vi "Periodic Task Hopper Control.vi"(8 "error in":errorcluster) -> ()   [LabVIEW 2016]
doc: "This VI runs in parallel to other tasks. It can contain as many user-defined periodic loops as you need. These can carry out PID or other sorts of timed response."
uses:
  Robot Global Data.vi
  HopperStates.ctl
  <vilib>/Rock Robotics/WPI/SafetyOutput/WPI_SafetyOutputConfigMenu.ctl
panel:
  in  "HighAutoDownSpeed":dbl=0.15
  in  "LowAutoDownSpeed":dbl=-0.15
  in  "HighAutoUpSpeed":dbl=-0.1
  in  "LowAutoUpSpeed":dbl=0.1
  in  "HighManualDownSpeed":dbl=0.15
  in  "LowManualDownSpeed":dbl=-0.15
  in  "HighManualUpSpeed":dbl=-0.1
  in  "LowManualUpSpeed":dbl=0.1
  in  "HighHopperMotorSpeed":dbl
  in  "LowHopperMotorSpeed":dbl
  in  "LDPhotoeyeOffTimerLimit":u32=200
  in  "LDPhotoeyeOnTimerLimit":u32=300
  in  "LDStartTimeOff":u32
  in  "LDPhotoeyeOnTimerDone":bool
  in  "LDStartTimeOn":u32
  in  "LDPhotoeyeOnTiming":bool
  in  "LDPhotoeyeOffTiming":bool
  in  "LUPhotoeyeOffTimerLimit":u32=200
  in  "LUPhotoeyeOnTimerLimit":u32=300
  in  "LUStartTimeOff":u32
  in  "LUPhotoeyeOnTimerDone":bool
  in  "LUStartTimeOn":u32
  in  "LUPhotoeyeOnTiming":bool
  in  "LUPhotoeyeOffTiming":bool
  in  "HDPhotoeyeOffTimerLimit":u32=200
  in  "HDPhotoeyeOnTimerLimit":u32=300
  in  "HDStartTimeOff":u32
  in  "HDPhotoeyeOnTimerDone":bool
  in  "HDStartTimeOn":u32
  in  "HDPhotoeyeOnTiming":bool
  in  "HDPhotoeyeOffTiming":bool
  in  "HUPhotoeyeOffTimerLimit":u32=200
  in  "HUPhotoeyeOnTimerLimit":u32=300
  in  "HUStartTimeOff":u32
  in  "HUPhotoeyeOnTimerDone":bool
  in  "HUStartTimeOn":u32
  in  "HUPhotoeyeOnTiming":bool
  in  "HUPhotoeyeOffTiming":bool
  # "High Side Up Photoeye"
  # "High Side Down Photoeye"
  # "Current Motor Speed"
  # "Manual Control Speed Settings"
  # "Low Side Up Photoeye"
  # "Low Side Down Photoeye"
  # "Automatic Control Speed Settings"
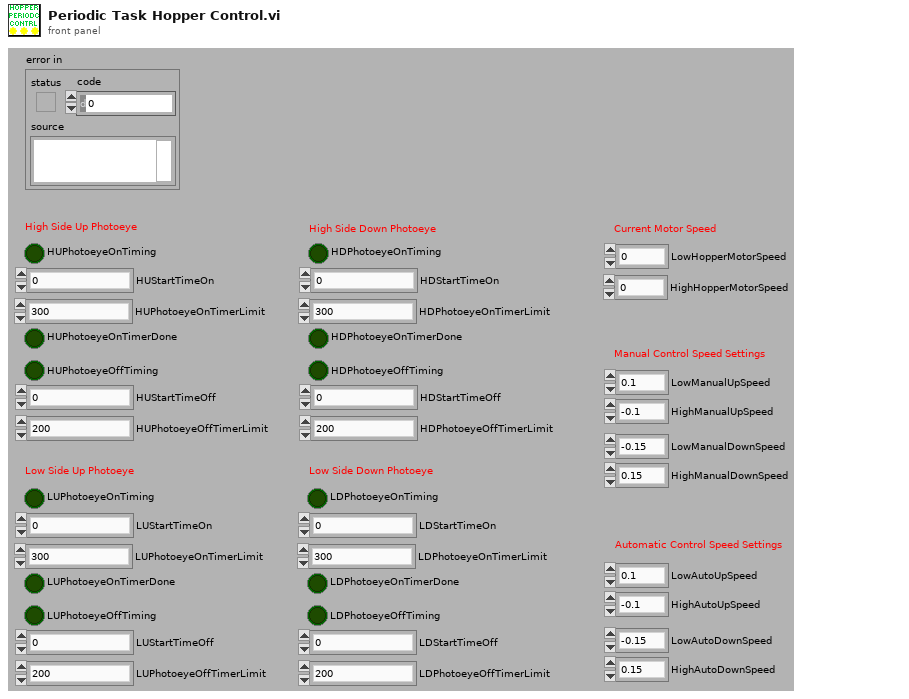
[diagram p1: front panel]
types:
  T1 = typedef "WPI_SafetyOutputConfigMenu.ctl" = enum16{"Enable", "Disable"}
  T2 = typedef "HopperStates.ctl" = enum16{"HopperIdle", "ManualRaiseHopper", "ManualLowerHopper", "AutoRaiseHopper", "AutoLowerHopper", "AtTop", "AtBottom"}
  T3 = typedef "WPI_MotorControlDeviceRef.ctl" = cluster{"DeviceStatus":errorcluster, "Type":T4, "PWM":cluster{"PWM Channel":T5, "DeadBand":T6}, "CAN":cluster{"Device Number":u8, "SetOutput VI Ref":variant, "GetOutput VI Ref":variant, "Enable VI Ref":variant, "Disable VI Ref":variant, "Data":variant}, "Invert":bool}
  T4 = typedef "WPI_MotorControlType.ctl" = enum16{"PWM", "CAN"}
  T5 = typedef "FPGA_DIOPWMChannel.ctl" = enum8{"PWM 0", "PWM 1", "PWM 2", "PWM 3", "PWM 4", "PWM 5", "PWM 6", "PWM 7", "PWM 8", "PWM 9", "PWM MXP 0", "PWM MXP 1", "PWM MXP 2", "PWM MXP 3", "PWM MXP 4", "PWM MXP 5", "PWM MXP 6", "PWM MXP 7", "PWM MXP 8", "PWM MXP 9", "Invalid"}
  T6 = typedef "WPI_PWMDeadband.ctl" = cluster{"Name":string, "maxPositivePwm":i32, "minPositivePwm":i32, "centerPwm":i32, "maxNegativePwm":i32, "minNegativePwm":i32, "angularRange":u16}
  T7 = typedef "WPI_DigitalInputDevRef.ctl" = cluster{"DevStatus":errorcluster, "DIO Channel":T8}
  T8 = typedef "FPGA_DIOChannel.ctl" = enum8{"DIO 0", "DIO 1", "DIO 2", "DIO 3", "DIO 4", "DIO 5", "DIO 6", "DIO 7", "DIO 8", "DIO 9", "DIO MXP 0", "DIO MXP 1", "DIO MXP 2", "DIO MXP 3", "DIO MXP 4", "DIO MXP 5", "DIO MXP 6", "DIO MXP 7", "DIO MXP 8", "DIO MXP 9", "DIO MXP 10", "DIO MXP 11", "DIO MXP 12", "DIO MXP 13", "DIO MXP 14", "DIO MXP 15", "SPI Port CS1", "SPI Port CS2", "SPI Port CS3", "SPI Port MISO", "SPI Port MOSI", "Invalid"}
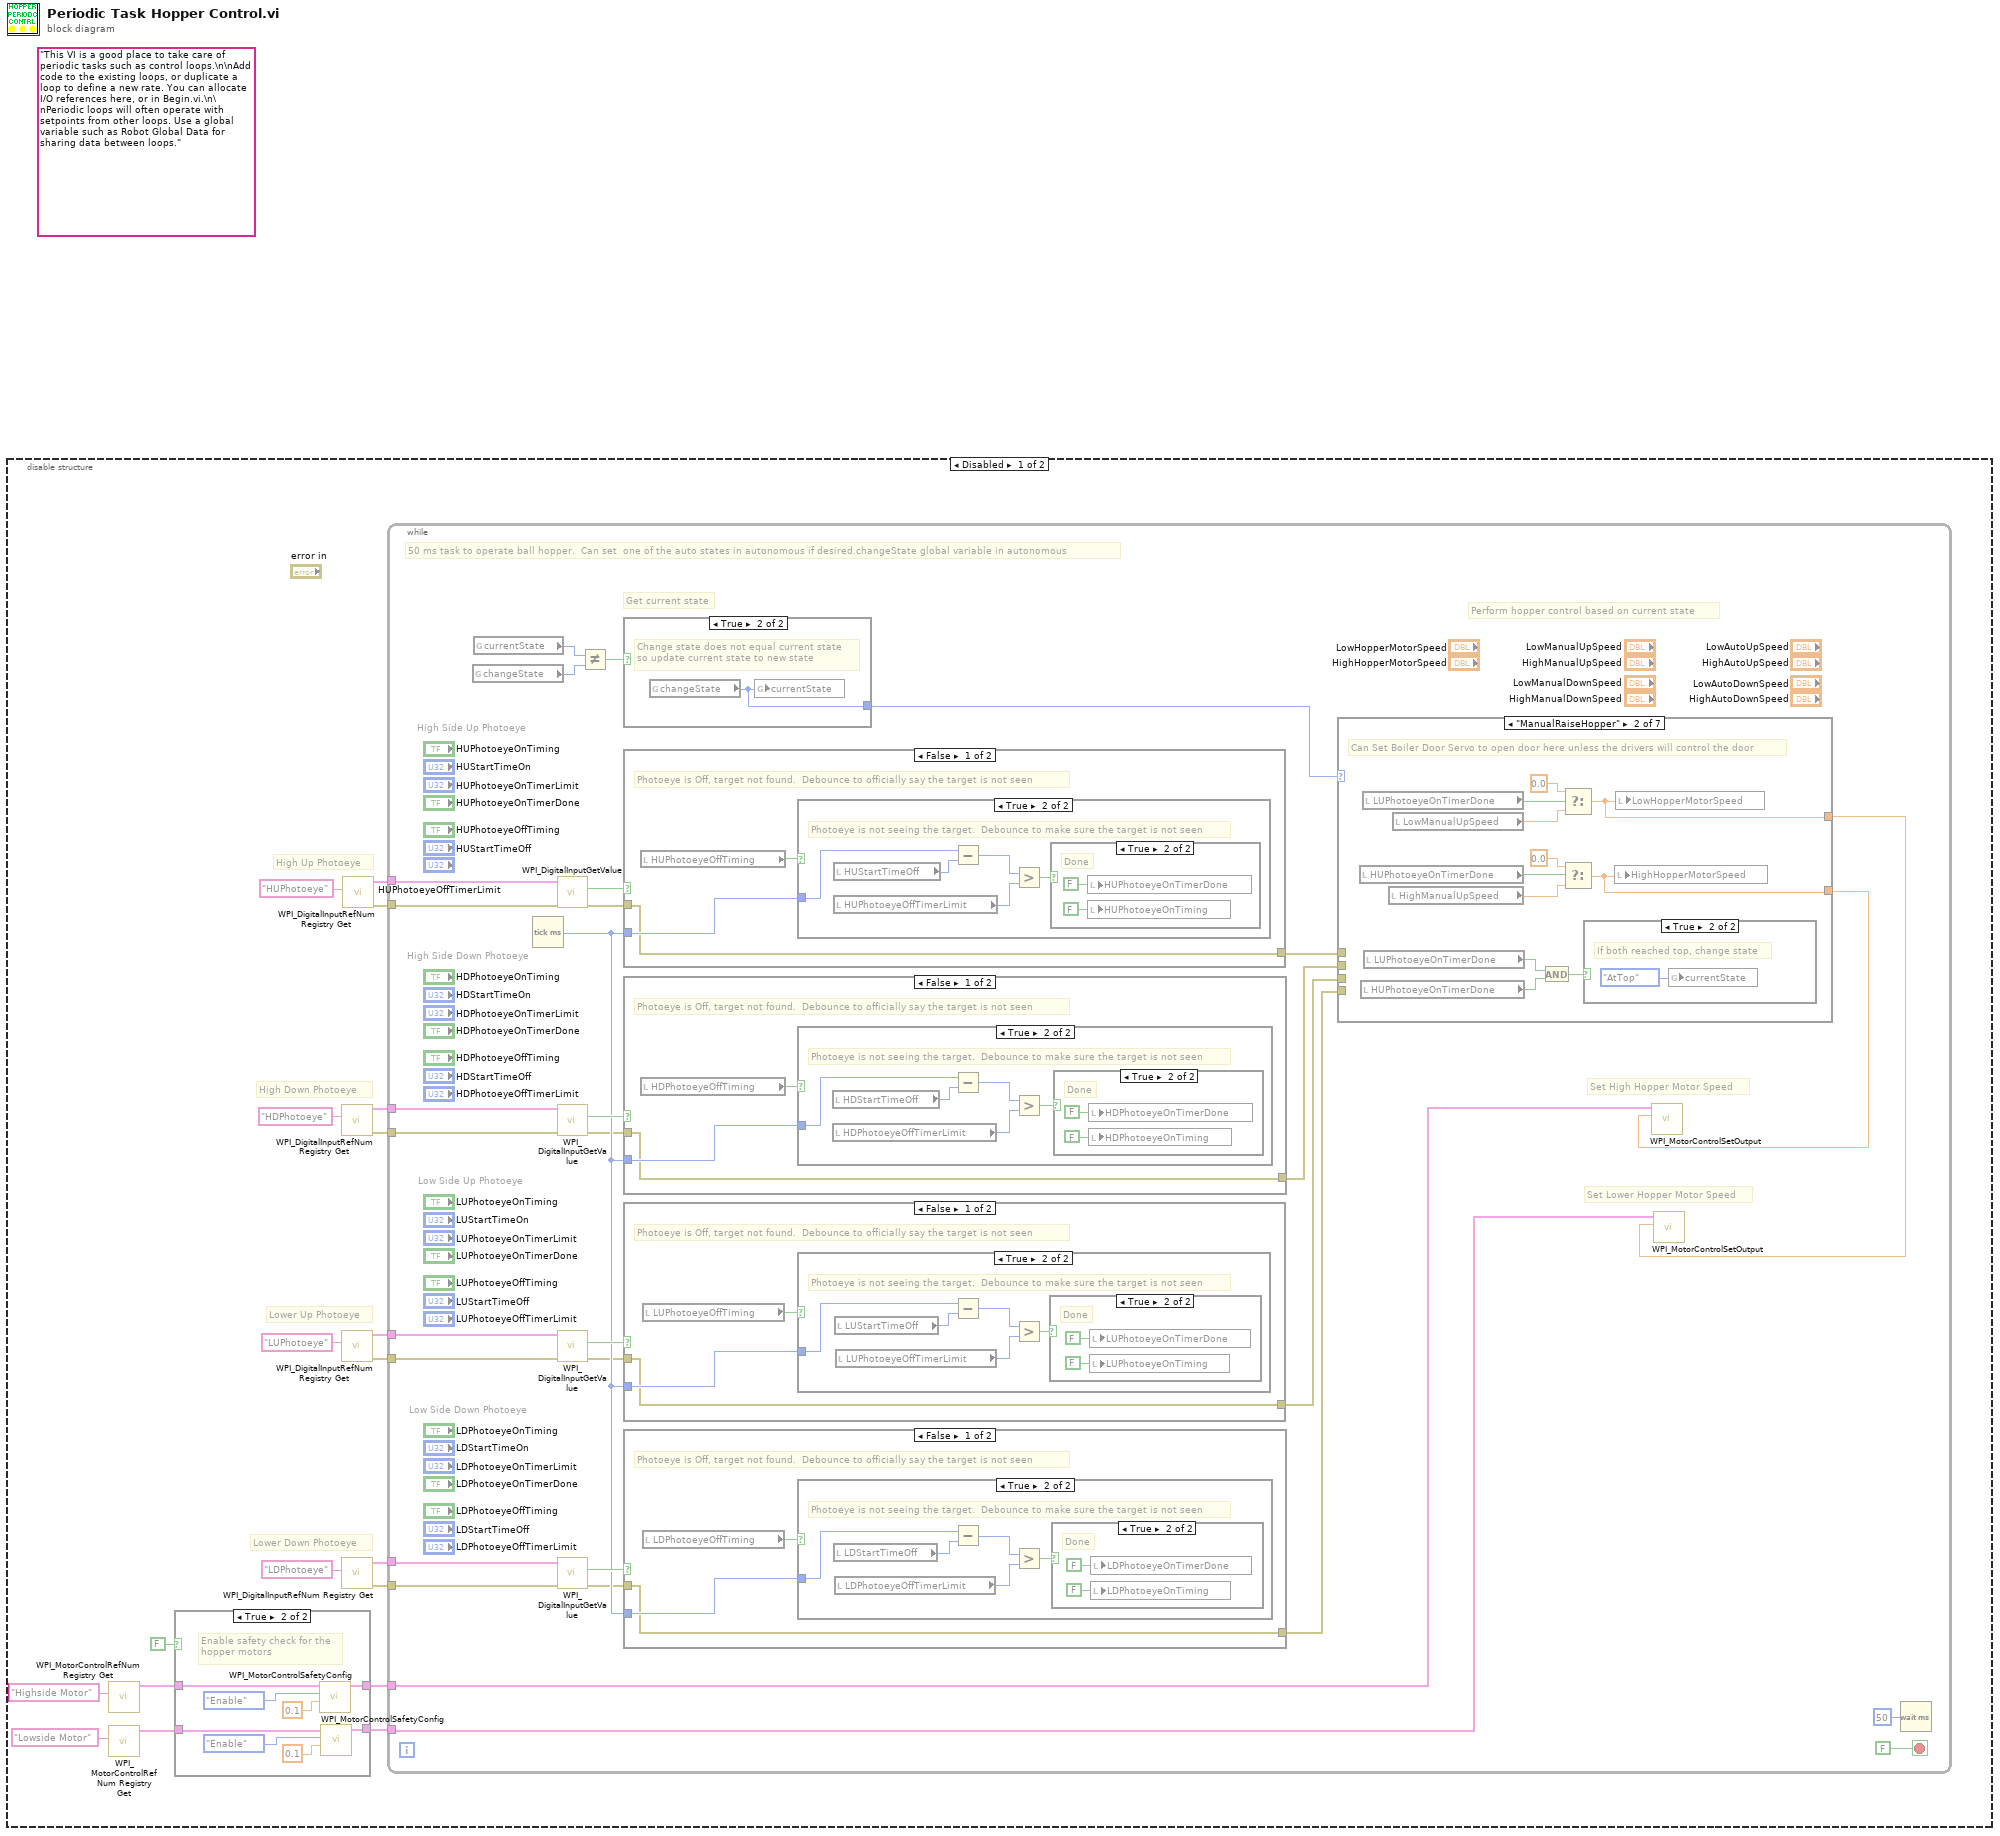
[diagram p0: block diagram]
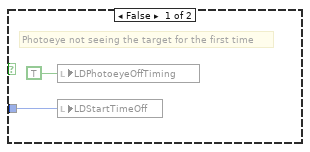
[diagram p3: hidden frame]
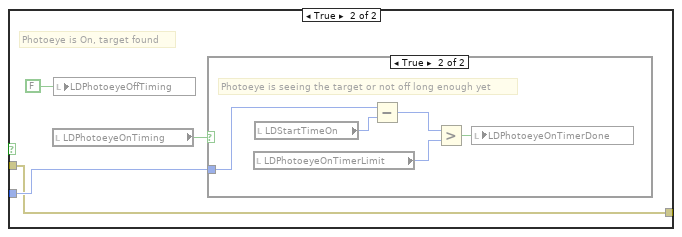
[diagram p5: hidden frame]
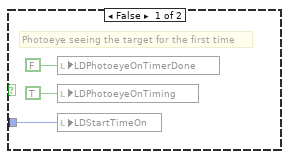
[diagram p6: hidden frame]
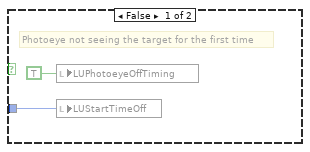
[diagram p7: hidden frame]
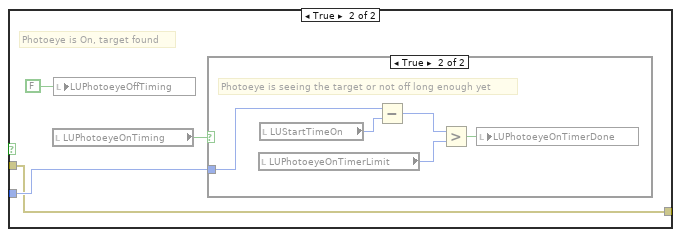
[diagram p9: hidden frame]
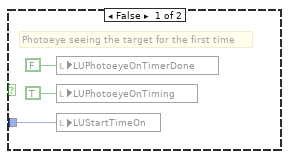
[diagram p10: hidden frame]
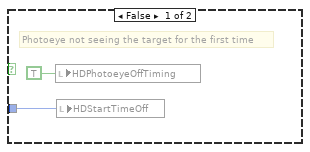
[diagram p11: hidden frame]
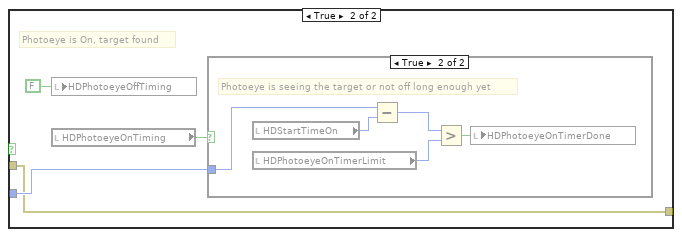
[diagram p13: hidden frame]
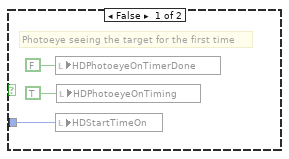
[diagram p14: hidden frame]
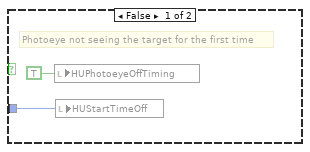
[diagram p15: hidden frame]
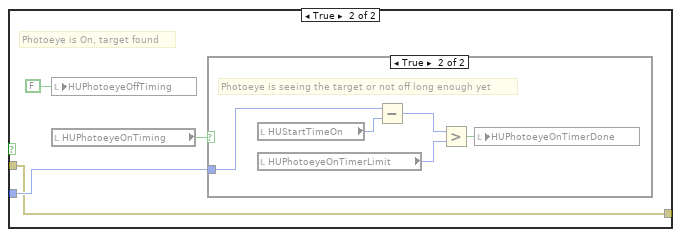
[diagram p17: hidden frame]
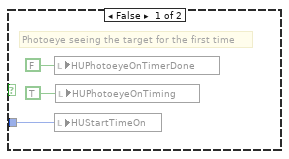
[diagram p18: hidden frame]
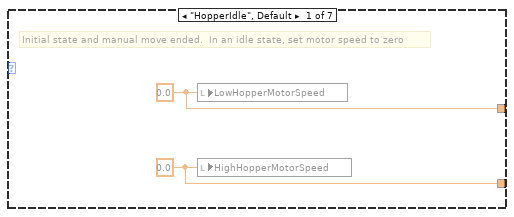
[diagram p19: hidden frame]
diagram:
  (unwired) "This VI is a good place to take care of periodic tasks such as control loops.\n\nAdd code to the existing loops, or duplicate a loop to define a new rate. You can allocate I/O references here, or in Begin.vi.\n\nPeriodic loops will often operate with setpoints from other loops. Use a global variable such as Robot Global Data for sharing data between loops."
  n1 = disable-structure shown="Disabled" {
    frame Disabled {
      # "Lower Down Photoeye"
      # "Lower Up Photoeye"
      # "High Down Photoeye"
      # "High Up Photoeye"
      n2 = call <vilib>:"WPI_MotorControlRefNum Registry Get.vi"("refnum name"="Highside Motor") -> ("MotorControlDevRef"=w5:T3)  [unwired: 9 in, 1 out]
      n3 = call <vilib>:"WPI_MotorControlRefNum Registry Get.vi"("refnum name"="Lowside Motor") -> ("MotorControlDevRef"=w3:T3)  [unwired: 9 in, 1 out]
      n4 = case shown="True" FALSE {
        tunnel: w5 -> [w21 w29]
        tunnel: [w21 w28] -> w4
        tunnel: w3 -> [w20 w27]
        tunnel: [w20 w26] -> w2
        frame False {
          # "Skip safety check since this\nVI loop should never be\nstarved"
        }
        frame True {
          # "Enable safety check for the\nhopper motors"
          n5 = call <vilib>:"WPI_MotorControlSafetyConfig.vi"("timeout (s)"=0.1, "mode"=WPI_SafetyOutputConfigMenu."Enable", "MotorControlDevRef"=w29) -> ("MotorControlDevRef"=w28:T3)  [unwired: 7 in, 1 out]
          n6 = call <vilib>:"WPI_MotorControlSafetyConfig.vi"("timeout (s)"=0.1, "mode"=WPI_SafetyOutputConfigMenu."Enable", "MotorControlDevRef"=w27) -> ("MotorControlDevRef"=w26:T3)  [unwired: 7 in, 1 out]
        }
      }
      n7 = call <vilib>:"WPI_DigitalInputRefNum Registry Get.vi"("refnum name"="HDPhotoeye") -> ("error out"=w8:errorcluster, "DigitalInputDevRef"=w9:T7)  [unwired: 9 in]
      n8 = call <vilib>:"WPI_DigitalInputRefNum Registry Get.vi"("refnum name"="LUPhotoeye") -> ("error out"=w10:errorcluster, "DigitalInputDevRef"=w11:T7)  [unwired: 9 in]
      n9 = call <vilib>:"WPI_DigitalInputRefNum Registry Get.vi"("refnum name"="LDPhotoeye") -> ("error out"=w12:errorcluster, "DigitalInputDevRef"=w13:T7)  [unwired: 9 in]
      n10 = call <vilib>:"WPI_DigitalInputRefNum Registry Get.vi"("refnum name"="HUPhotoeye") -> ("error out"=w17:errorcluster, "DigitalInputDevRef"=w18:T7)  [unwired: 9 in]
      n11 = while {
        tunnel: w18 -> [w41]
        tunnel: w17 -> [w40]
        tunnel: w9 -> [w39]
        tunnel: w8 -> [w38]
        tunnel: w11 -> [w37]
        tunnel: w10 -> [w36]
        tunnel: w13 -> [w35]
        tunnel: w12 -> [w34]
        tunnel: w2 -> [w30]
        tunnel: w4 -> [w31]
        stop <- FALSE stop-if-true
        # "Low Side Down Photoeye"
        # "Low Side Up Photoeye"
        # "High Side Down Photoeye"
        # "High Side Up Photoeye"
        # "Set Lower Hopper Motor Speed"
        # "Set High Hopper Motor Speed"
        # "Get current state"
        # "Perform hopper control based on current state"
        # "50 ms task to operate ball hopper.  Can set  one of the auto states in autonomous if desired.changeState global variable in autonomous"
        n12 = global read "Robot Global Data.vi" "changeState"() -> (w57:T2)
        n13 = global read "Robot Global Data.vi" "currentState"() -> (w58:T2)
        n14 = Tick Count (ms)() -> (millisecond timer value=w50:u32)
        n15 = call <vilib>:"WPI_DigitalInputGetValue.vi"("error in (no error)"=w40, "DigitalInputDevRef"=w41) -> ("error out"=w48:errorcluster, "Value"=w54:bool)  [unwired: 7 in, 1 out]
        n16 = call <vilib>:"WPI_DigitalInputGetValue.vi"("error in (no error)"=w38, "DigitalInputDevRef"=w39) -> ("error out"=w47:errorcluster, "Value"=w53:bool)  [unwired: 7 in, 1 out]
        n17 = call <vilib>:"WPI_DigitalInputGetValue.vi"("error in (no error)"=w36, "DigitalInputDevRef"=w37) -> ("error out"=w46:errorcluster, "Value"=w52:bool)  [unwired: 7 in, 1 out]
        n18 = call <vilib>:"WPI_DigitalInputGetValue.vi"("error in (no error)"=w34, "DigitalInputDevRef"=w35) -> ("error out"=w49:errorcluster, "Value"=w51:bool)  [unwired: 7 in, 1 out]
        n19 = Not Equal?(x=w58, y=w57) -> (x != y?=w56:bool)
        n20 = case shown="True" w56 {
          tunnel: [w211 w212] -> w55
          frame False {
            # "Change state equals current state \nso keep current state"
            n21 = global read "Robot Global Data.vi" "currentState"() -> (w211:T2)
          }
          frame True {
            # "Change state does not equal current state \nso update current state to new state"
            n22 = global read "Robot Global Data.vi" "changeState"() -> (w212:T2)
            n23 = global write "Robot Global Data.vi" "currentState"(w212) -> ()
          }
        }
        n24 = case shown="False" w54 {
          tunnel: w50 -> [w134 w146]
          tunnel: w48 -> [w133 w145]
          tunnel: [w133 w145] -> w45
          frame False {
            # "Photoeye is Off, target not found.  Debounce to officially say the target is not seen"
            n25 = local read "HUPhotoeyeOffTiming"() -> (w135:bool)
            n26 = case shown="True" w135 {
              tunnel: w134 -> [w137 w141]
              frame False {
                # "Photoeye not seeing the target for the first time"
                n27 = local write "HUPhotoeyeOffTiming"(TRUE ("PhotoeyeOffTiming")) -> ()
                n28 = local write "HUStartTimeOff"(w137) -> ()
              }
              frame True {
                # "Photoeye is not seeing the target.  Debounce to make sure the target is not seen"
                n29 = local read "HUStartTimeOff"() -> (w140:u32)
                n30 = local read "HUPhotoeyeOffTimerLimit"() -> (w139:u32)
                n31 = Subtract(x=w141, y=w140) -> (x-y=w142:u32)
                n32 = Greater?(x=w142, y=w139) -> (0:w138:bool)
                n33 = case shown="True" w138 {
                  frame False {
                    # "Waiting for Off to time out"
                  }
                  frame True {
                    # "Done"
                    n34 = local write "HUPhotoeyeOnTimerDone"(FALSE ("HUPhotoeyeOnTimerDone")) -> ()
                    n35 = local write "HUPhotoeyeOnTiming"(FALSE ("HUPhotoeyeOnTiming")) -> ()
                  }
                }
              }
            }
          }
          frame True {
            # "Photoeye is On, target found"
            n36 = local write "HUPhotoeyeOffTiming"(FALSE ("PhotoeyeOffTiming")) -> ()
            n37 = local read "HUPhotoeyeOnTiming"() -> (w147:bool)
            n38 = case shown="True" w147 {
              tunnel: w146 -> [w151 w156]
              frame False {
                # "Photoeye seeing the target for the first time"
                n39 = local write "HUPhotoeyeOnTimerDone"(FALSE ("PhotoeyeOnTimerDone")) -> ()
                n40 = local write "HUStartTimeOn"(w151) -> ()
                n41 = local write "HUPhotoeyeOnTiming"(TRUE ("PhotoeyeOnTiming")) -> ()
              }
              frame True {
                # "Photoeye is seeing the target or not off long enough yet"
                n42 = local read "HUStartTimeOn"() -> (w155:u32)
                n43 = local read "HUPhotoeyeOnTimerLimit"() -> (w153:u32)
                n44 = Subtract(x=w156, y=w155) -> (x-y=w154:u32)
                n45 = Greater?(x=w154, y=w153) -> (0:w152:bool)
                n46 = local write "HUPhotoeyeOnTimerDone"(w152) -> ()
              }
            }
          }
        }
        n47 = case shown="False" w53 {
          tunnel: w50 -> [w110 w122]
          tunnel: w47 -> [w109 w121]
          tunnel: [w109 w121] -> w44
          frame False {
            # "Photoeye is Off, target not found.  Debounce to officially say the target is not seen"
            n48 = local read "HDPhotoeyeOffTiming"() -> (w111:bool)
            n49 = case shown="True" w111 {
              tunnel: w110 -> [w113 w117]
              frame False {
                # "Photoeye not seeing the target for the first time"
                n50 = local write "HDPhotoeyeOffTiming"(TRUE ("PhotoeyeOffTiming")) -> ()
                n51 = local write "HDStartTimeOff"(w113) -> ()
              }
              frame True {
                # "Photoeye is not seeing the target.  Debounce to make sure the target is not seen"
                n52 = local read "HDStartTimeOff"() -> (w116:u32)
                n53 = local read "HDPhotoeyeOffTimerLimit"() -> (w115:u32)
                n54 = Subtract(x=w117, y=w116) -> (x-y=w118:u32)
                n55 = Greater?(x=w118, y=w115) -> (0:w114:bool)
                n56 = case shown="True" w114 {
                  frame False {
                    # "Waiting for Off to time out"
                  }
                  frame True {
                    # "Done"
                    n57 = local write "HDPhotoeyeOnTimerDone"(FALSE ("HDPhotoeyeOnTimerDone")) -> ()
                    n58 = local write "HDPhotoeyeOnTiming"(FALSE ("HDPhotoeyeOnTiming")) -> ()
                  }
                }
              }
            }
          }
          frame True {
            # "Photoeye is On, target found"
            n59 = local write "HDPhotoeyeOffTiming"(FALSE ("PhotoeyeOffTiming")) -> ()
            n60 = local read "HDPhotoeyeOnTiming"() -> (w123:bool)
            n61 = case shown="True" w123 {
              tunnel: w122 -> [w127 w132]
              frame False {
                # "Photoeye seeing the target for the first time"
                n62 = local write "HDPhotoeyeOnTimerDone"(FALSE ("PhotoeyeOnTimerDone")) -> ()
                n63 = local write "HDStartTimeOn"(w127) -> ()
                n64 = local write "HDPhotoeyeOnTiming"(TRUE ("PhotoeyeOnTiming")) -> ()
              }
              frame True {
                # "Photoeye is seeing the target or not off long enough yet"
                n65 = local read "HDStartTimeOn"() -> (w131:u32)
                n66 = local read "HDPhotoeyeOnTimerLimit"() -> (w129:u32)
                n67 = Subtract(x=w132, y=w131) -> (x-y=w130:u32)
                n68 = Greater?(x=w130, y=w129) -> (0:w128:bool)
                n69 = local write "HDPhotoeyeOnTimerDone"(w128) -> ()
              }
            }
          }
        }
        n70 = case shown="False" w52 {
          tunnel: w50 -> [w86 w98]
          tunnel: w46 -> [w85 w97]
          tunnel: [w85 w97] -> w43
          frame False {
            # "Photoeye is Off, target not found.  Debounce to officially say the target is not seen"
            n71 = local read "LUPhotoeyeOffTiming"() -> (w87:bool)
            n72 = case shown="True" w87 {
              tunnel: w86 -> [w89 w93]
              frame False {
                # "Photoeye not seeing the target for the first time"
                n73 = local write "LUPhotoeyeOffTiming"(TRUE ("PhotoeyeOffTiming")) -> ()
                n74 = local write "LUStartTimeOff"(w89) -> ()
              }
              frame True {
                # "Photoeye is not seeing the target.  Debounce to make sure the target is not seen"
                n75 = local read "LUStartTimeOff"() -> (w92:u32)
                n76 = local read "LUPhotoeyeOffTimerLimit"() -> (w91:u32)
                n77 = Subtract(x=w93, y=w92) -> (x-y=w94:u32)
                n78 = Greater?(x=w94, y=w91) -> (0:w90:bool)
                n79 = case shown="True" w90 {
                  frame False {
                    # "Waiting for Off to time out"
                  }
                  frame True {
                    # "Done"
                    n80 = local write "LUPhotoeyeOnTimerDone"(FALSE ("LUPhotoeyeOnTimerDone")) -> ()
                    n81 = local write "LUPhotoeyeOnTiming"(FALSE ("LUPhotoeyeOnTiming")) -> ()
                  }
                }
              }
            }
          }
          frame True {
            # "Photoeye is On, target found"
            n82 = local read "LUPhotoeyeOnTiming"() -> (w99:bool)
            n83 = local write "LUPhotoeyeOffTiming"(FALSE ("PhotoeyeOffTiming")) -> ()
            n84 = case shown="True" w99 {
              tunnel: w98 -> [w103 w108]
              frame False {
                # "Photoeye seeing the target for the first time"
                n85 = local write "LUPhotoeyeOnTimerDone"(FALSE ("PhotoeyeOnTimerDone")) -> ()
                n86 = local write "LUPhotoeyeOnTiming"(TRUE ("PhotoeyeOnTiming")) -> ()
                n87 = local write "LUStartTimeOn"(w103) -> ()
              }
              frame True {
                # "Photoeye is seeing the target or not off long enough yet"
                n88 = local read "LUPhotoeyeOnTimerLimit"() -> (w105:u32)
                n89 = local read "LUStartTimeOn"() -> (w107:u32)
                n90 = Subtract(x=w108, y=w107) -> (x-y=w106:u32)
                n91 = Greater?(x=w106, y=w105) -> (0:w104:bool)
                n92 = local write "LUPhotoeyeOnTimerDone"(w104) -> ()
              }
            }
          }
        }
        n93 = case shown="False" w51 {
          tunnel: w50 -> [w62 w74]
          tunnel: w49 -> [w61 w73]
          tunnel: [w61 w73] -> w42
          frame False {
            # "Photoeye is Off, target not found.  Debounce to officially say the target is not seen"
            n94 = local read "LDPhotoeyeOffTiming"() -> (w63:bool)
            n95 = case shown="True" w63 {
              tunnel: w62 -> [w65 w69]
              frame False {
                # "Photoeye not seeing the target for the first time"
                n96 = local write "LDPhotoeyeOffTiming"(TRUE ("PhotoeyeOffTiming")) -> ()
                n97 = local write "LDStartTimeOff"(w65) -> ()
              }
              frame True {
                # "Photoeye is not seeing the target.  Debounce to make sure the target is not seen"
                n98 = local read "LDStartTimeOff"() -> (w68:u32)
                n99 = local read "LDPhotoeyeOffTimerLimit"() -> (w67:u32)
                n100 = Subtract(x=w69, y=w68) -> (x-y=w70:u32)
                n101 = Greater?(x=w70, y=w67) -> (0:w66:bool)
                n102 = case shown="True" w66 {
                  frame False {
                    # "Waiting for Off to time out"
                  }
                  frame True {
                    # "Done"
                    n103 = local write "LDPhotoeyeOnTimerDone"(FALSE ("LDPhotoeyeOnTimerDone")) -> ()
                    n104 = local write "LDPhotoeyeOnTiming"(FALSE ("LDPhotoeyeOnTiming")) -> ()
                  }
                }
              }
            }
          }
          frame True {
            # "Photoeye is On, target found"
            n105 = local read "LDPhotoeyeOnTiming"() -> (w75:bool)
            n106 = local write "LDPhotoeyeOffTiming"(FALSE ("PhotoeyeOffTiming")) -> ()
            n107 = case shown="True" w75 {
              tunnel: w74 -> [w79 w84]
              frame False {
                # "Photoeye seeing the target for the first time"
                n108 = local write "LDPhotoeyeOnTimerDone"(FALSE ("PhotoeyeOnTimerDone")) -> ()
                n109 = local write "LDPhotoeyeOnTiming"(TRUE ("PhotoeyeOnTiming")) -> ()
                n110 = local write "LDStartTimeOn"(w79) -> ()
              }
              frame True {
                # "Photoeye is seeing the target or not off long enough yet"
                n111 = local read "LDPhotoeyeOnTimerLimit"() -> (w81:u32)
                n112 = local read "LDStartTimeOn"() -> (w83:u32)
                n113 = Subtract(x=w84, y=w83) -> (x-y=w82:u32)
                n114 = Greater?(x=w82, y=w81) -> (0:w80:bool)
                n115 = local write "LDPhotoeyeOnTimerDone"(w80) -> ()
              }
            }
          }
        }
        n116 = case shown="\"ManualRaiseHopper\"" w55 {
          tunnel: w45 -> [_ _ _ _ _ _ _]
          tunnel: w44 -> [_ _ _ _ _ _ _]
          tunnel: w43 -> [_ _ _ _ _ _ _]
          tunnel: w42 -> [_ _ _ _ _ _ _]
          tunnel: [w158 w160 w172 w184 w196 w207 w210] -> w33
          tunnel: [w157 w159 w171 w183 w195 w208 w209] -> w32
          frame "HopperIdle", Default {
            w157 = 0.0 ("HighHopperMotorSpeed")
            w158 = 0.0 ("LowHopperMotorSpeed")
            # "Initial state and manual move ended.  In an idle state, set motor speed to zero"
            n117 = local write "LowHopperMotorSpeed"(w158) -> ()
            n118 = local write "HighHopperMotorSpeed"(w157) -> ()
          }
          frame "ManualRaiseHopper" {
            # "Can Set Boiler Door Servo to open door here unless the drivers will control the door"
            n119 = local read "HUPhotoeyeOnTimerDone"() -> (w165:bool)
            n120 = local read "HUPhotoeyeOnTimerDone"() -> (w161:bool)
            n121 = local read "LUPhotoeyeOnTimerDone"() -> (w169:bool)
            n122 = local read "LUPhotoeyeOnTimerDone"() -> (w162:bool)
            n123 = local read "HighManualUpSpeed"() -> (w164:dbl)
            n124 = local read "LowManualUpSpeed"() -> (w167:dbl)
            n125 = And(x=w162, y=w161) -> (x .and. y?=w163:bool)
            n126 = Select(t=0.0, s=w169, f=w167) -> (s? t:f=w160:dbl)
            n127 = Select(t=0.0, s=w165, f=w164) -> (s? t:f=w159:dbl)
            n128 = case shown="True" w163 {
              frame False {
                # "Do Nothing"
              }
              frame True {
                # "If both reached top, change state"
                n129 = global write "Robot Global Data.vi" "currentState"(HopperStates."AtTop" ("currentState")) -> ()
              }
            }
            n130 = local write "HighHopperMotorSpeed"(w159) -> ()
            n131 = local write "LowHopperMotorSpeed"(w160) -> ()
          }
          frame "ManualLowerHopper" {
            # "Can Set Boiler Door Servo to close door here unless the drivers will control the door"
            n132 = local read "HDPhotoeyeOnTimerDone"() -> (w178:bool)
            n133 = local read "HDPhotoeyeOnTimerDone"() -> (w173:bool)
            n134 = local read "LDPhotoeyeOnTimerDone"() -> (w179:bool)
            n135 = local read "LDPhotoeyeOnTimerDone"() -> (w174:bool)
            n136 = local read "HighManualDownSpeed"() -> (w176:dbl)
            n137 = local read "LowManualDownSpeed"() -> (w177:dbl)
            n138 = And(x=w174, y=w173) -> (x .and. y?=w175:bool)
            n139 = Select(t=0.0, s=w179, f=w177) -> (s? t:f=w172:dbl)
            n140 = Select(t=0.0, s=w178, f=w176) -> (s? t:f=w171:dbl)
            n141 = case shown="True" w175 {
              frame False {
                # "Do Nothing"
              }
              frame True {
                # "If both reached bottom, change state"
                n142 = global write "Robot Global Data.vi" "currentState"(HopperStates."AtBottom" ("currentState")) -> ()
              }
            }
            n143 = local write "HighHopperMotorSpeed"(w171) -> ()
            n144 = local write "LowHopperMotorSpeed"(w172) -> ()
          }
          frame "AutoRaiseHopper" {
            # "Can Set Boiler Door Servo to open door here unless the drivers will control the door"
            n145 = local read "HUPhotoeyeOnTimerDone"() -> (w191:bool)
            n146 = local read "HUPhotoeyeOnTimerDone"() -> (w185:bool)
            n147 = local read "LUPhotoeyeOnTimerDone"() -> (w190:bool)
            n148 = local read "LUPhotoeyeOnTimerDone"() -> (w186:bool)
            n149 = local read "HighAutoUpSpeed"() -> (w188:dbl)
            n150 = local read "LowAutoUpSpeed"() -> (w189:dbl)
            n151 = And(x=w186, y=w185) -> (x .and. y?=w187:bool)
            n152 = Select(t=0.0, s=w190, f=w189) -> (s? t:f=w184:dbl)
            n153 = Select(t=0.0, s=w191, f=w188) -> (s? t:f=w183:dbl)
            n154 = case shown="True" w187 {
              frame False {
                # "Do Nothing"
              }
              frame True {
                # "If both reached top, change state"
                n155 = global write "Robot Global Data.vi" "currentState"(HopperStates."AtTop" ("currentState")) -> ()
              }
            }
            n156 = local write "HighHopperMotorSpeed"(w183) -> ()
            n157 = local write "LowHopperMotorSpeed"(w184) -> ()
          }
          frame "AutoLowerHopper" {
            # "Can Set Boiler Door Servo to close door here unless the drivers will control the door"
            n158 = local read "HDPhotoeyeOnTimerDone"() -> (w203:bool)
            n159 = local read "HDPhotoeyeOnTimerDone"() -> (w198:bool)
            n160 = local read "LDPhotoeyeOnTimerDone"() -> (w202:bool)
            n161 = local read "LDPhotoeyeOnTimerDone"() -> (w197:bool)
            n162 = local read "HighAutoDownSpeed"() -> (w200:dbl)
            n163 = local read "LowAutoDownSpeed"() -> (w199:dbl)
            n164 = And(x=w197, y=w198) -> (x .and. y?=w201:bool)
            n165 = Select(t=0.0, s=w202, f=w199) -> (s? t:f=w196:dbl)
            n166 = Select(t=0.0, s=w203, f=w200) -> (s? t:f=w195:dbl)
            n167 = case shown="True" w201 {
              frame False {
                # "Do Nothing"
              }
              frame True {
                # "If both reached bottom, change state"
                n168 = global write "Robot Global Data.vi" "currentState"(HopperStates."AtBottom" ("currentState")) -> ()
              }
            }
            n169 = local write "HighHopperMotorSpeed"(w195) -> ()
            n170 = local write "LowHopperMotorSpeed"(w196) -> ()
          }
          frame "AtTop" {
            w208 = 0.0 ("HighHopperMotorSpeed")
            w207 = 0.0 ("LowHopperMotorSpeed")
            # "Reached the top.  In an idle state, set motor speed to zero"
            n171 = local write "LowHopperMotorSpeed"(w207) -> ()
            n172 = local write "HighHopperMotorSpeed"(w208) -> ()
          }
          frame "AtBottom" {
            w209 = 0.0 ("HighHopperMotorSpeed")
            w210 = 0.0 ("LowHopperMotorSpeed")
            # "Reached the bottom.  In an idle state, set motor speed to zero"
            n173 = local write "LowHopperMotorSpeed"(w210) -> ()
            n174 = local write "HighHopperMotorSpeed"(w209) -> ()
          }
        }
        n175 = call <vilib>:"WPI_MotorControlSetOutput.vi"("Output"=w32, "MotorControlDevRef"=w31) -> ()  [unwired: 7 in, 3 out]
        n176 = call <vilib>:"WPI_MotorControlSetOutput.vi"("Output"=w33, "MotorControlDevRef"=w30) -> ()  [unwired: 7 in, 3 out]
        n177 = Wait (ms)(milliseconds to wait=u32 50) -> ()  [unwired: 1 out]
      }
    }
    frame Enabled {
    }
  }
